vi "Add wtaer usage.vi"() -> (3 "Numeric":dbl)   [LabVIEW 2019]
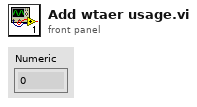
[diagram p1: front panel]
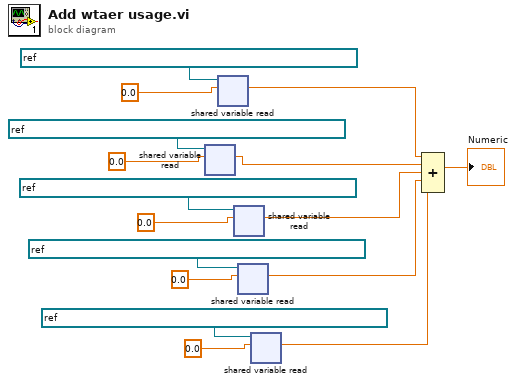
[diagram p0: block diagram]
diagram:
  n1 = shared-variable-read(refnum<k21> "ni.var.psp://z004551/CDL0100 ReadTags/Rinse2_Flow_Total" ("shared variable refnum in"), 0.0) -> (w13:dbl)  [unwired: 1 in, 3 out]
  n2 = shared-variable-read(refnum<k21> "ni.var.psp://z004551/CDL0100 ReadTags/Rinse1_Flow_Total" ("shared variable refnum in"), 0.0) -> (w12:dbl)  [unwired: 1 in, 3 out]
  n3 = shared-variable-read(refnum<k21> "ni.var.psp://z004551/CDL0100 ReadTags/Rinse3_Flow_Total" ("shared variable refnum in"), 0.0) -> (w14:dbl)  [unwired: 1 in, 3 out]
  n4 = shared-variable-read(refnum<k21> "ni.var.psp://z004551/CDL0100 ReadTags/Rinse4_Flow_Total" ("shared variable refnum in"), 0.0) -> (w15:dbl)  [unwired: 1 in, 3 out]
  n5 = shared-variable-read(refnum<k21> "ni.var.psp://z004551/CDL0100 ReadTags/BAS_DI_RunningTot" ("shared variable refnum in"), 0.0) -> (w1:dbl)  [unwired: 1 in, 3 out]
  n6 = Compound Arithmetic op=ADD(w12, w13, w14, w15, w1) -> (→"Numeric":dbl)
